vi "start acquisition.vi"(8 "error in (no error)":errorcluster, 9 "Image Type":T1=1 items=["Grayscale (U8)", "Grayscale (I16)", "Grayscale (SGL)", "Complex (CSG)", "RGB (U32)", "HSL (U32)", "RGB (U64)", "Grayscale (U16)"], 10 "Camera Name":T2, 11 "IMAQdx Cam in":refnum<class "IMAQdx Cam.lvclass">) -> (0 "error out":errorcluster, 2 "Event Registration Refnum":refnum<event-registration>, 3 "IMAQdx Cam out":refnum<class "IMAQdx Cam.lvclass">)   [LabVIEW 2020, in "IMAQdx Cam.lvclass"]
uses:
  IMAQdx Cam.lvclass
  <vilib>/userdefined/High Color/IMAQdx.ctl
  <vilib>/vision/driver/IMAQdx.llb/IMAQdx Camera Control Mode.ctl
  <vilib>/vision/driver/IMAQdx.llb/IMAQdx Acquisition Mode.ctl
  IMAQdx Cam.lvclass/IMAQdx Cam.ctl
  <vilib>/vision/driver/NI_Vision_Acquisition_Software.lvlib
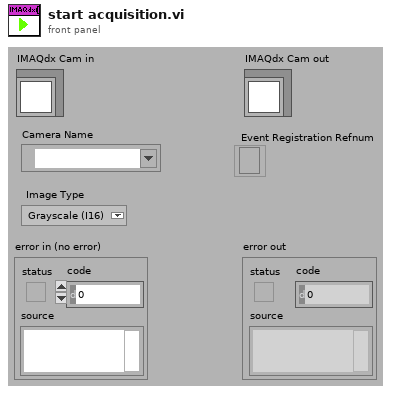
[diagram p1: front panel]
types:
  T1 = typedef "Image Type" = u32
  T2 = typedef "IMAQdx.ctl" = refnum<k21>
  T3 = typedef "NI_Vision_Acquisition_Software.lvlib/IMAQdx Acquisition Mode.ctl" = enum32{"One Shot", "Continuous"}
  T4 = typedef "NI_Vision_Acquisition_Software.lvlib/IMAQdx Camera Control Mode.ctl" = enum32{"Controller", "Listener"}
  T5 = typedef "IMAQ Image.ctl" = refnum<image>
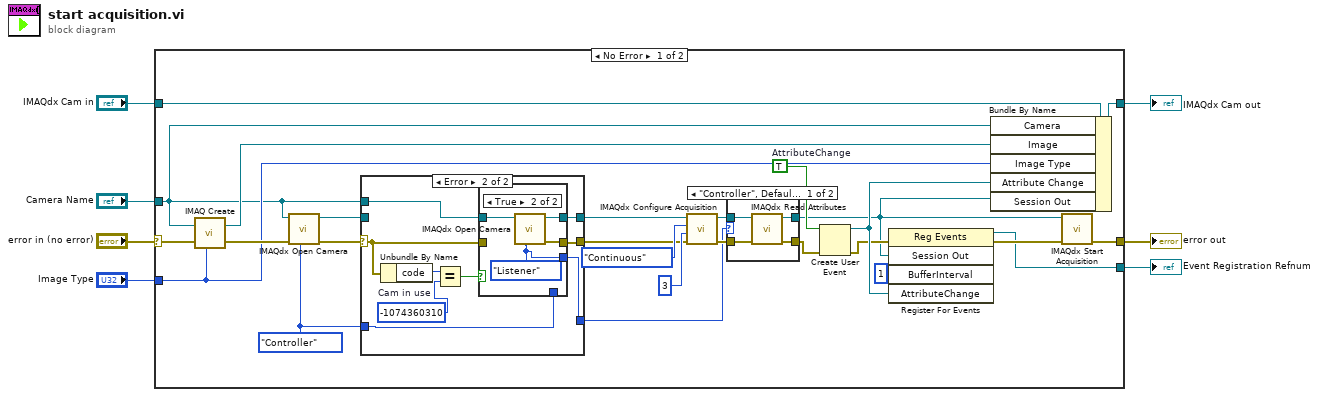
[diagram p0: block diagram]
diagram:
  n1 = case shown="No Error" "error in (no error)" {
    selector: "error in (no error)" -> [w28 w60]
    tunnel: [w31 w60] -> w6
    tunnel: [w29 w59] -> w4
    tunnel: "IMAQdx Cam in" -> [w30 w59]
    tunnel: "Camera Name" -> [w18 _]
    tunnel: [w25 _] -> w1
    tunnel: "Image Type" -> [w22 _]
    frame No Error {
      w24 = TRUE  # AttributeChange
      w9 = IMAQdx_Camera_Control_Mode."Controller" ("Camera Control Mode")
      n2 = call "IMAQ Create"("Image Name"=w18, "Image Type"=w22, "error in (no error)"=w28) -> ("New Image"=w19:T5, "error out"=w27:errorcluster)  [unwired: 1 in, 1 out]
      n3 = call <vilib>:"IMAQdx Open Camera.vi"("Camera Control Mode"=w9, "error in"=w27, "Session In"=w18) -> ("error out"=w20:errorcluster, "Session Out"=w33:T2)  [unwired: 7 out]
      n4 = case shown="Error" w20 {
        selector: w20 -> [w41 w46]
        tunnel: w33 -> [w42 _]
        tunnel: [w42 w49] -> w11
        tunnel: [w41 w48] -> w13
        tunnel: w18 -> [_ w45]
        tunnel: w9 -> [w40 w43]
        tunnel: [w40 w44] -> w8
        frame No Error {
        }
        frame Error {
          w50 = -1074360310  # Cam in use
          n5 = Unbundle By Name(w46) -> ("code"=w51:i32)
          n6 = Equal?(x=w51, y=w50) -> (x = y?=w47:bool)
          n7 = case shown="True" w47 {
            tunnel: w45 -> [w53 w58]
            tunnel: [w53 w56] -> w49
            tunnel: [w54 w57] -> w48
            tunnel: w46 -> [w54 _]
            tunnel: [w52 w55] -> w44
            tunnel: w43 -> [w52 _]
            frame False {
            }
            frame True {
              w55 = IMAQdx_Camera_Control_Mode."Listener" ("Camera Control Mode")
              n8 = call <vilib>:"IMAQdx Open Camera.vi"("Camera Control Mode"=w55, "Session In"=w58) -> ("error out"=w57:errorcluster, "Session Out"=w56:T2)  [unwired: 1 in, 7 out]
            }
          }
        }
      }
      n9 = call <vilib>:"IMAQdx Configure Acquisition.vi"("error in"=w13, "Number of Buffers"=u32 3, "Continuous?"=IMAQdx_Acquisition_Mode."Continuous", "Session In"=w11) -> ("error out"=w17:errorcluster, "Session Out"=w16:T2)  [unwired: 6 out]
      n10 = case shown="\"Controller\", Default" w8 {
        tunnel: w17 -> [w37 w38]
        tunnel: w16 -> [w36 w39]
        tunnel: [w35 w38] -> w12
        tunnel: [w34 w39] -> w10
        frame "Controller", Default {
          n11 = call <vilib>:"IMAQdx Read Attributes.vi"("error in"=w37, "Session In"=w36) -> ("error out"=w35:errorcluster, "Session Out"=w34:T2)  [unwired: 8 in]
        }
        frame "Listener" {
        }
      }
      n12 = Create User Event(user event datatype=w24, error in=w12) -> (user event=w23:refnum<user-event>, error out=w21:errorcluster)
      n13 = register-events(error in=w21, w10, u32 1 ("BufferInterval"), w23) -> (reference out=w25:refnum<event-registration>, error out=w32:errorcluster)  [unwired: 1 in]
      n14 = Bundle By Name(cluster=w30, "Camera"=w18, "Image"=w19, "Image Type"=w22, "Attribute Change"=w23, "Session Out"=w10) -> (w29:refnum<class "IMAQdx Cam.lvclass">)
      n15 = call <vilib>:"IMAQdx Start Acquisition.vi"("error in"=w32, "Session In"=w10) -> ("error out"=w31:errorcluster)  [unwired: 9 out]
    }
    frame Error {
    }
  }
  "error out" <- w6
  "IMAQdx Cam out" <- w4
  "Event Registration Refnum" <- w1
